vi "ControlMotorDefinePostionParam.vi"() -> (1 "位置信息":T2)   [LabVIEW 2018]
panel:
  out "准直光焦点":cluster{"控制电机":T1, "位置":dbl}[](array[cluster])
  out "光谱":cluster{"控制电机":T1, "位置":dbl}[](array[cluster])
  out "功率":cluster{"控制电机":T1, "位置":dbl}[](array[cluster])
  out "能量":cluster{"控制电机":T1, "位置":dbl}[](array[cluster])
  out "偏振":cluster{"控制电机":T1, "位置":dbl}[](array[cluster])
  out "时间波形":cluster{"控制电机":T1, "位置":dbl}[](array[cluster])
  out "近场相机":cluster{"控制电机":T1, "位置":dbl}[](array[cluster])
  out "远场相机":cluster{"控制电机":T1, "位置":dbl}[](array[cluster])
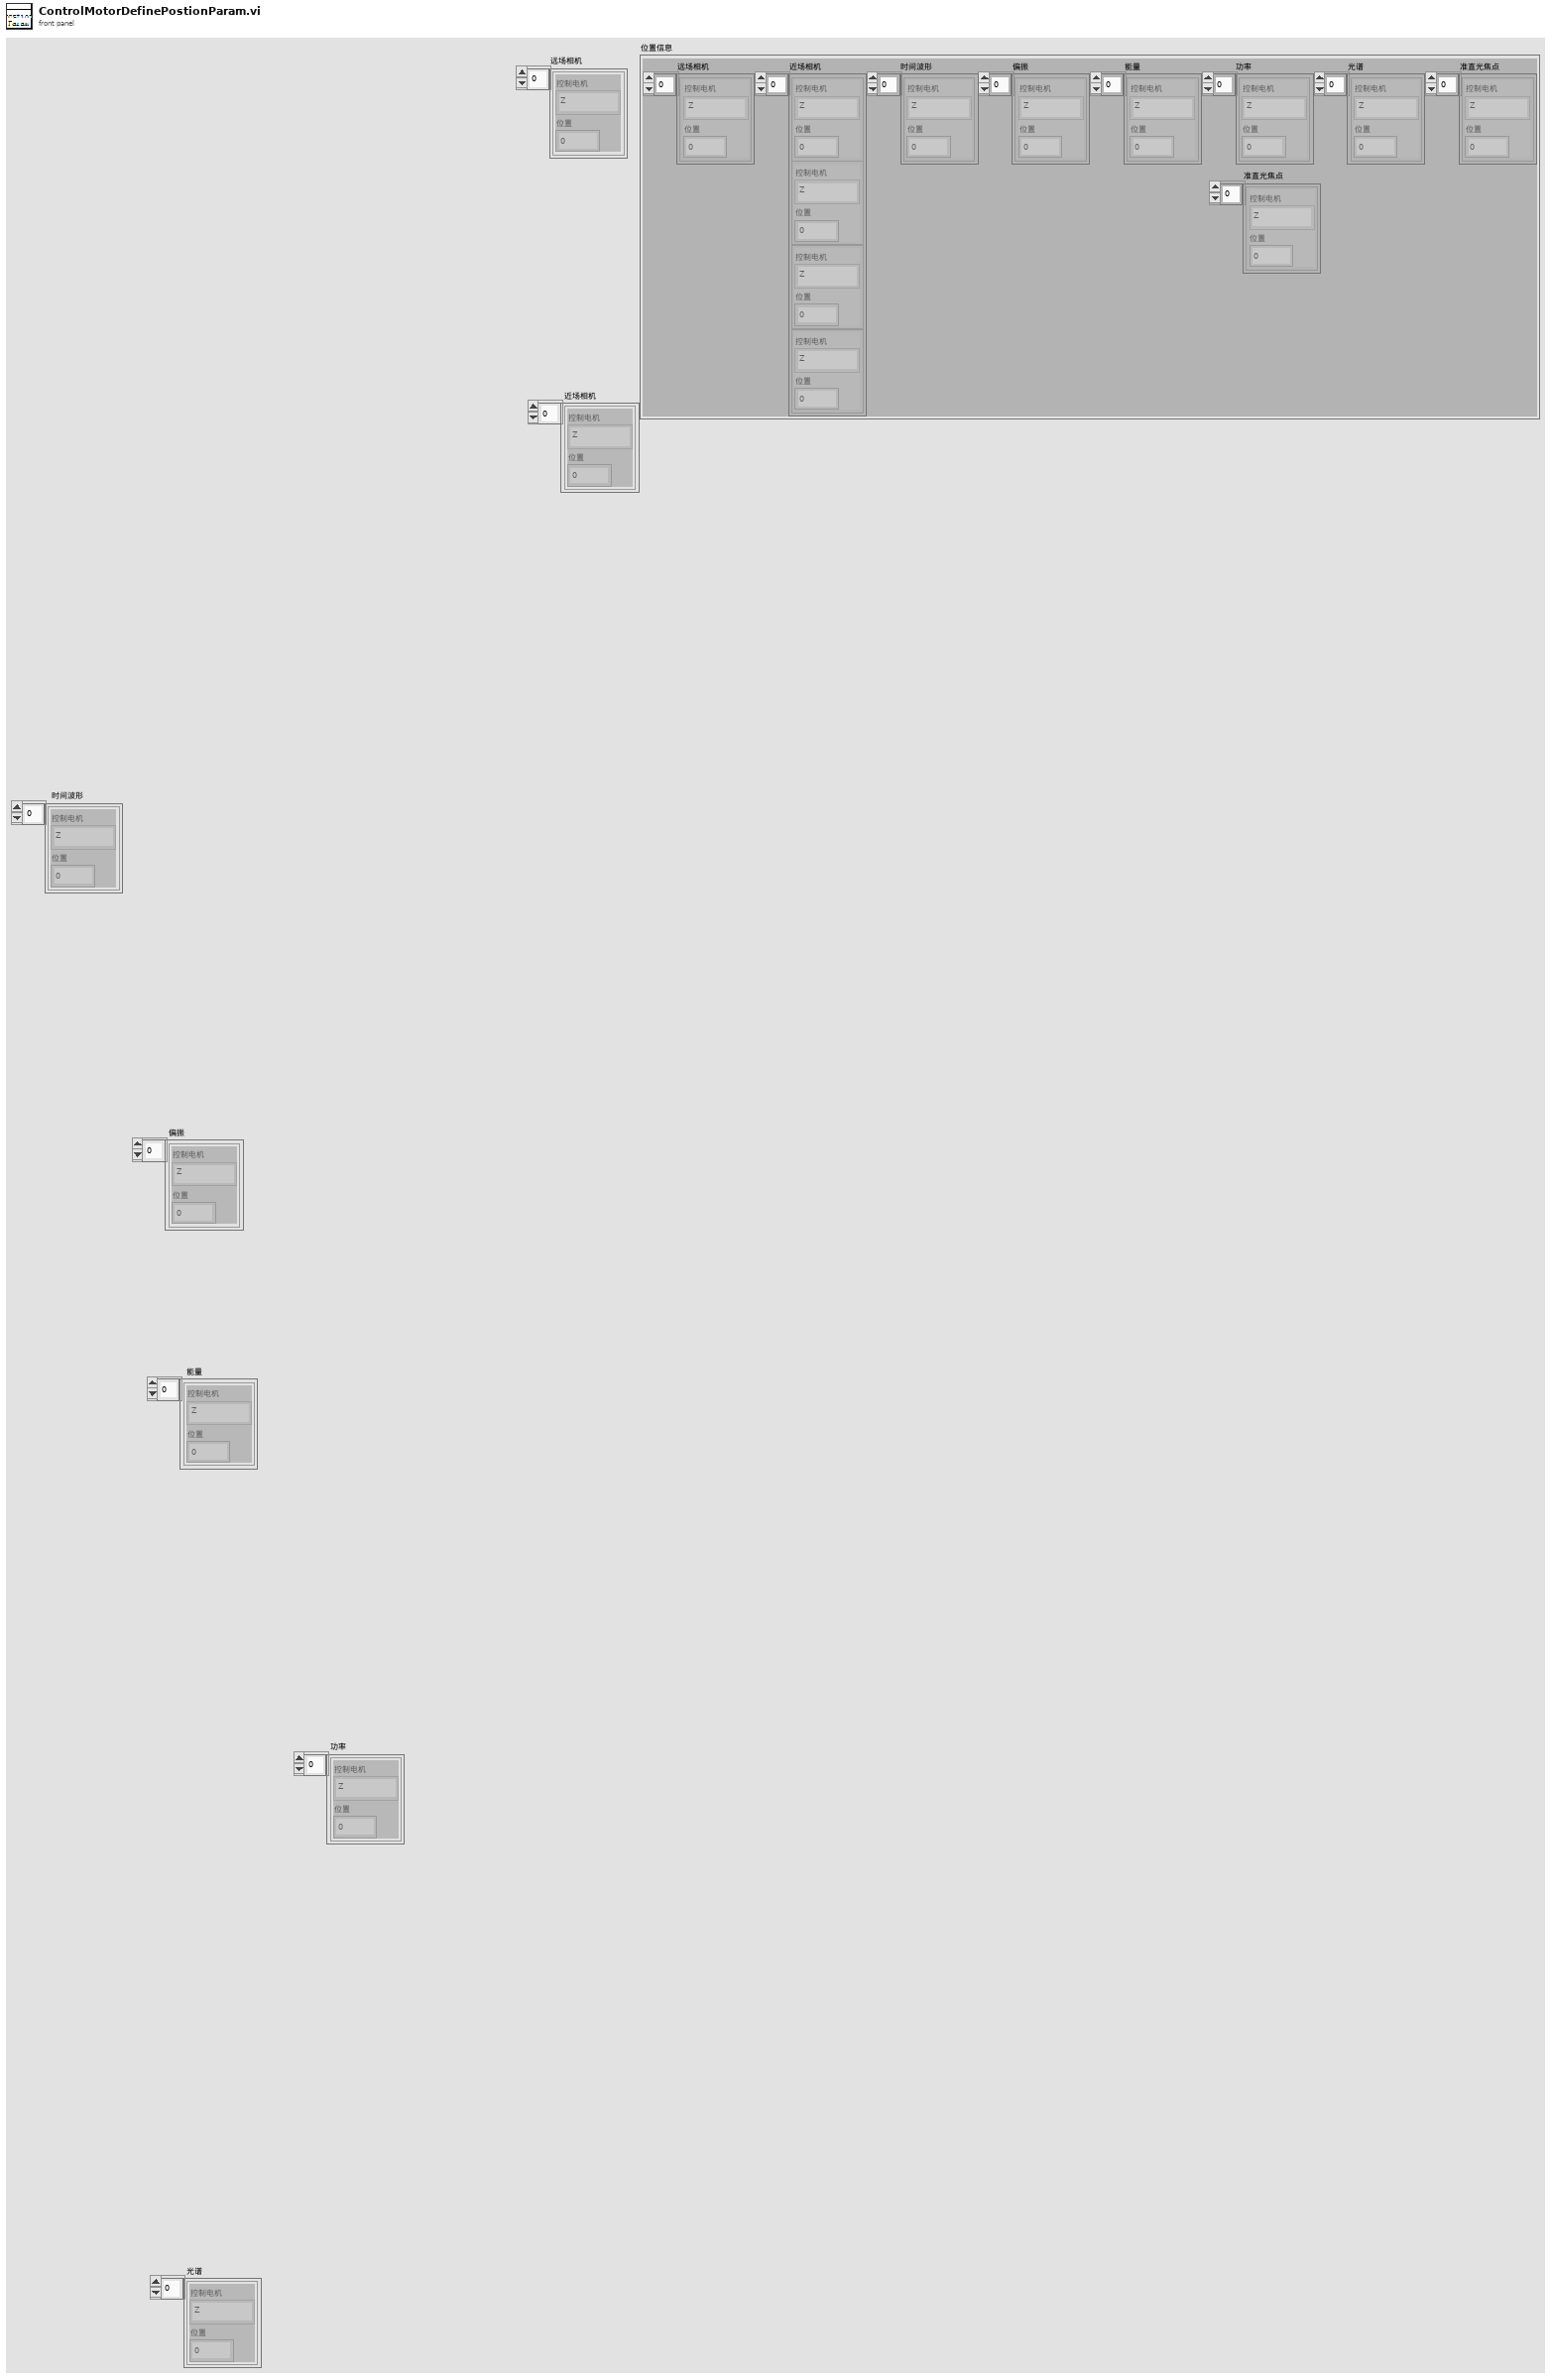
[diagram p1: front panel]
types:
  T1 = typedef "控制电机枚举器.ctl" = enum16{"Z", "Y", "X", "发散角", "俯仰", "旋转"}
  T2 = cluster{"远场相机":cluster{"控制电机":T1, "位置":dbl}[], "近场相机":cluster{"控制电机":T1, "位置":dbl}[], "时间波形":cluster{"控制电机":T1, "位置":dbl}[], "偏振":cluster{"控制电机":T1, "位置":dbl}[], "能量":cluster{"控制电机":T1, "位置":dbl}[], "功率":cluster{"控制电机":T1, "位置":dbl}[], "光谱":cluster{"控制电机":T1, "位置":dbl}[], "准直光焦点":cluster{"控制电机":T1, "位置":dbl}[]}
  T3 = cluster{cluster{"控制电机":T1, "位置":dbl}[], cluster{"控制电机":T1, "位置":dbl}[], cluster{"控制电机":T1, "位置":dbl}[], cluster{"控制电机":T1, "位置":dbl}[], cluster{"控制电机":T1, "位置":dbl}[], cluster{"控制电机":T1, "位置":dbl}[], cluster{"控制电机":T1, "位置":dbl}[], cluster{"控制电机":T1, "位置":dbl}[]}
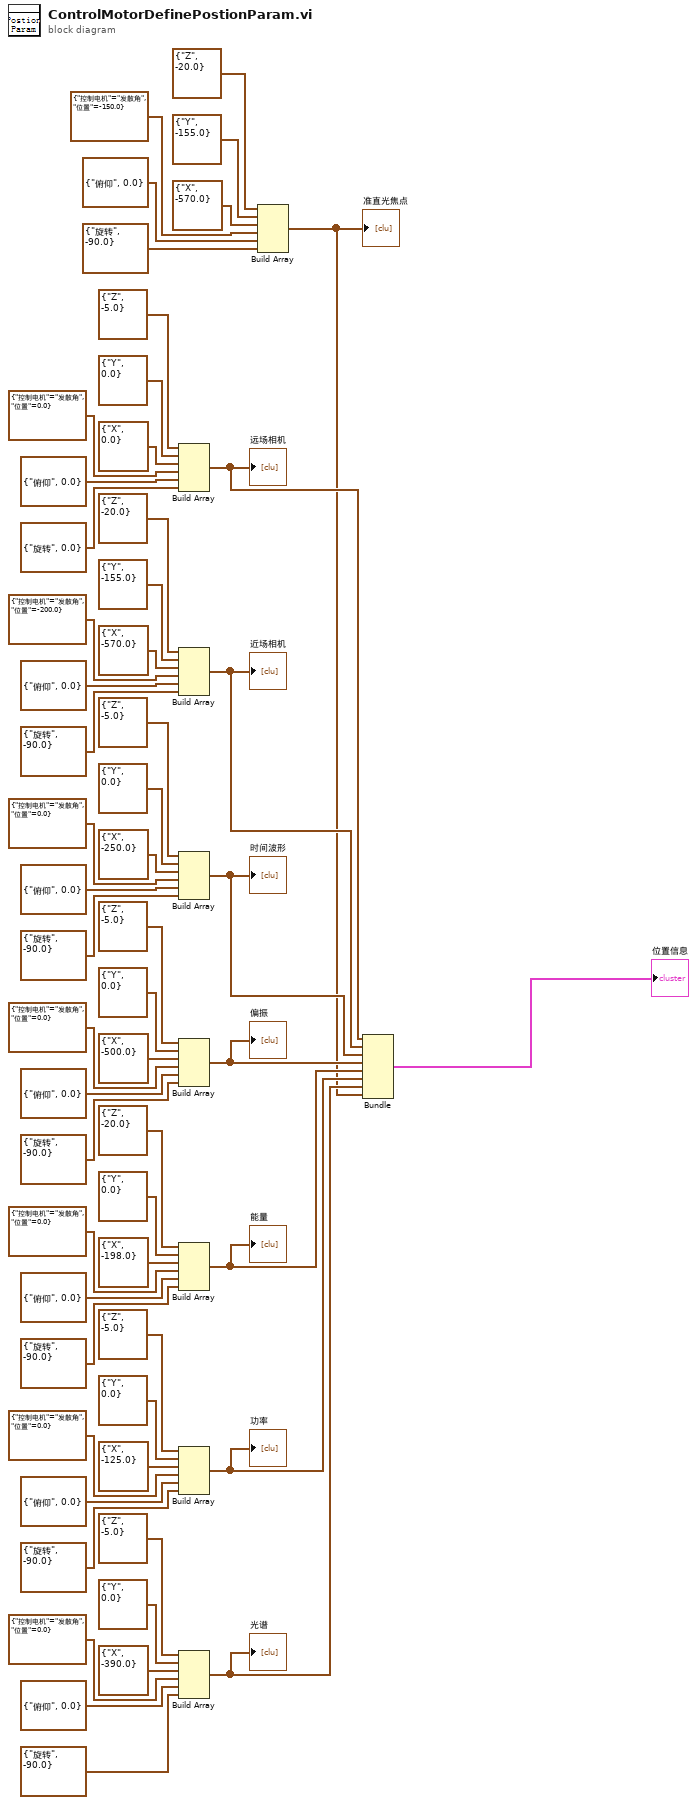
[diagram p0: block diagram]
diagram:
  n1 = Build Array(cluster{"控制电机":T1, "位置":dbl} {"控制电机"=enum."Z", "位置"=-5.0} ("元素"), cluster{"控制电机":T1, "位置":dbl} {"控制电机"=enum."Y", "位置"=0.0} ("元素"), cluster{"控制电机":T1, "位置":dbl} {"控制电机"=enum."X", "位置"=0.0} ("元素"), cluster{"控制电机":T1, "位置":dbl} {"控制电机"=enum."发散角", "位置"=0.0} ("元素"), cluster{"控制电机":T1, "位置":dbl} {"控制电机"=enum."俯仰", "位置"=0.0} ("元素"), cluster{"控制电机":T1, "位置":dbl} {"控制电机"=enum."旋转", "位置"=0.0} ("元素")) -> (w15:cluster{"控制电机":T1, "位置":dbl}[])
  "远场相机" <- w15
  n2 = Build Array(cluster{"控制电机":T1, "位置":dbl} {"控制电机"=enum."Z", "位置"=-20.0} ("元素"), cluster{"控制电机":T1, "位置":dbl} {"控制电机"=enum."Y", "位置"=-155.0} ("元素"), cluster{"控制电机":T1, "位置":dbl} {"控制电机"=enum."X", "位置"=-570.0} ("元素"), cluster{"控制电机":T1, "位置":dbl} {"控制电机"=enum."发散角", "位置"=-200.0} ("元素"), cluster{"控制电机":T1, "位置":dbl} {"控制电机"=enum."俯仰", "位置"=0.0} ("元素"), cluster{"控制电机":T1, "位置":dbl} {"控制电机"=enum."旋转", "位置"=-90.0} ("元素")) -> (w14:cluster{"控制电机":T1, "位置":dbl}[])
  "近场相机" <- w14
  n3 = Build Array(cluster{"控制电机":T1, "位置":dbl} {"控制电机"=enum."Z", "位置"=-5.0} ("元素"), cluster{"控制电机":T1, "位置":dbl} {"控制电机"=enum."Y", "位置"=0.0} ("元素"), cluster{"控制电机":T1, "位置":dbl} {"控制电机"=enum."X", "位置"=-250.0} ("元素"), cluster{"控制电机":T1, "位置":dbl} {"控制电机"=enum."发散角", "位置"=0.0} ("元素"), cluster{"控制电机":T1, "位置":dbl} {"控制电机"=enum."俯仰", "位置"=0.0} ("元素"), cluster{"控制电机":T1, "位置":dbl} {"控制电机"=enum."旋转", "位置"=-90.0} ("元素")) -> (w13:cluster{"控制电机":T1, "位置":dbl}[])
  "时间波形" <- w13
  n4 = Build Array(cluster{"控制电机":T1, "位置":dbl} {"控制电机"=enum."Z", "位置"=-5.0} ("元素"), cluster{"控制电机":T1, "位置":dbl} {"控制电机"=enum."Y", "位置"=0.0} ("元素"), cluster{"控制电机":T1, "位置":dbl} {"控制电机"=enum."X", "位置"=-500.0} ("元素"), cluster{"控制电机":T1, "位置":dbl} {"控制电机"=enum."发散角", "位置"=0.0} ("元素"), cluster{"控制电机":T1, "位置":dbl} {"控制电机"=enum."俯仰", "位置"=0.0} ("元素"), cluster{"控制电机":T1, "位置":dbl} {"控制电机"=enum."旋转", "位置"=-90.0} ("元素")) -> (w12:cluster{"控制电机":T1, "位置":dbl}[])
  "偏振" <- w12
  n5 = Build Array(cluster{"控制电机":T1, "位置":dbl} {"控制电机"=enum."Z", "位置"=-20.0} ("元素"), cluster{"控制电机":T1, "位置":dbl} {"控制电机"=enum."Y", "位置"=0.0} ("元素"), cluster{"控制电机":T1, "位置":dbl} {"控制电机"=enum."X", "位置"=-198.0} ("元素"), cluster{"控制电机":T1, "位置":dbl} {"控制电机"=enum."发散角", "位置"=0.0} ("元素"), cluster{"控制电机":T1, "位置":dbl} {"控制电机"=enum."俯仰", "位置"=0.0} ("元素"), cluster{"控制电机":T1, "位置":dbl} {"控制电机"=enum."旋转", "位置"=-90.0} ("元素")) -> (w11:cluster{"控制电机":T1, "位置":dbl}[])
  "能量" <- w11
  n6 = Build Array(cluster{"控制电机":T1, "位置":dbl} {"控制电机"=enum."Z", "位置"=-5.0} ("元素"), cluster{"控制电机":T1, "位置":dbl} {"控制电机"=enum."Y", "位置"=0.0} ("元素"), cluster{"控制电机":T1, "位置":dbl} {"控制电机"=enum."X", "位置"=-125.0} ("元素"), cluster{"控制电机":T1, "位置":dbl} {"控制电机"=enum."发散角", "位置"=0.0} ("元素"), cluster{"控制电机":T1, "位置":dbl} {"控制电机"=enum."俯仰", "位置"=0.0} ("元素"), cluster{"控制电机":T1, "位置":dbl} {"控制电机"=enum."旋转", "位置"=-90.0} ("元素")) -> (w10:cluster{"控制电机":T1, "位置":dbl}[])
  "功率" <- w10
  n7 = Build Array(cluster{"控制电机":T1, "位置":dbl} {"控制电机"=enum."Z", "位置"=-5.0} ("元素"), cluster{"控制电机":T1, "位置":dbl} {"控制电机"=enum."Y", "位置"=0.0} ("元素"), cluster{"控制电机":T1, "位置":dbl} {"控制电机"=enum."X", "位置"=-390.0} ("元素"), cluster{"控制电机":T1, "位置":dbl} {"控制电机"=enum."发散角", "位置"=0.0} ("元素"), cluster{"控制电机":T1, "位置":dbl} {"控制电机"=enum."俯仰", "位置"=0.0} ("元素"), cluster{"控制电机":T1, "位置":dbl} {"控制电机"=enum."旋转", "位置"=-90.0} ("元素")) -> (w9:cluster{"控制电机":T1, "位置":dbl}[])
  "光谱" <- w9
  n8 = Build Array(cluster{"控制电机":T1, "位置":dbl} {"控制电机"=enum."Z", "位置"=-20.0} ("元素"), cluster{"控制电机":T1, "位置":dbl} {"控制电机"=enum."Y", "位置"=-155.0} ("元素"), cluster{"控制电机":T1, "位置":dbl} {"控制电机"=enum."X", "位置"=-570.0} ("元素"), cluster{"控制电机":T1, "位置":dbl} {"控制电机"=enum."发散角", "位置"=-150.0} ("元素"), cluster{"控制电机":T1, "位置":dbl} {"控制电机"=enum."俯仰", "位置"=0.0} ("元素"), cluster{"控制电机":T1, "位置":dbl} {"控制电机"=enum."旋转", "位置"=-90.0} ("元素")) -> (w2:cluster{"控制电机":T1, "位置":dbl}[])
  "准直光焦点" <- w2
  n9 = Bundle(w15, w14, w13, w12, w11, w10, w9, w2) -> (→"位置信息":T3)  [unwired: 1 in]
